vi "Message encoder.vi"(8 "error in (no error)":errorcluster, 10 "Data":variant, 11 "Kasli Writer in":refnum<class "Kasli Writer.lvclass">) -> (0 "error out":errorcluster, 2 "Message encoded":string, 3 "Kasli Writer out":refnum<class "Kasli Writer.lvclass">)   [LabVIEW 2020, in "CIRCUS_uServices.lvlib" / "Kasli Listener and Writer.lvlib" / "Kasli Writer.lvclass"]
uses:
  Kasli Writer.lvclass
  TALOS/TALOS_PPL.lvlibp
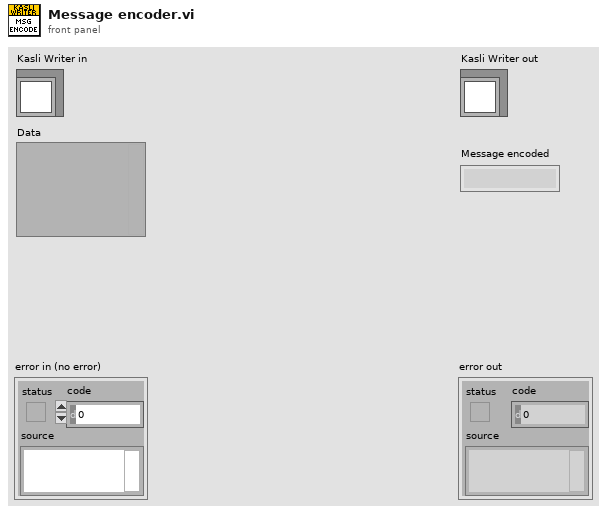
[diagram p1: front panel]
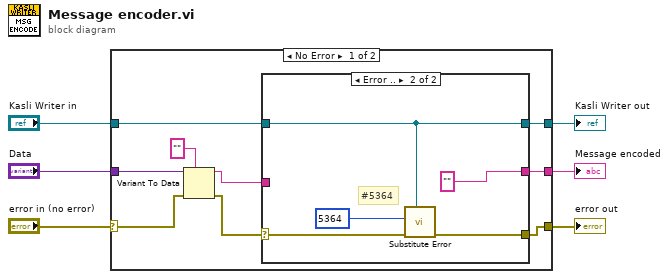
[diagram p0: block diagram]
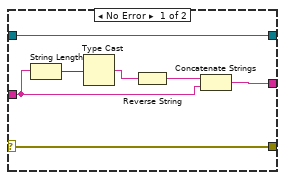
[diagram p2: hidden frame]
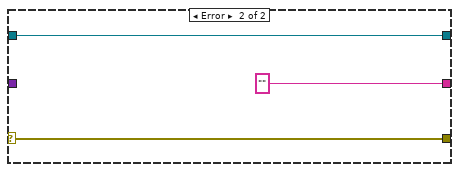
[diagram p3: hidden frame]
diagram:
  n1 = case shown="No Error" "error in (no error)" {
    selector: "error in (no error)" -> [w13 w28]
    tunnel: "Data" -> [w15 _]
    tunnel: [w7 ""] -> w5
    tunnel: [w8 w28] -> w3
    tunnel: "Kasli Writer in" -> [w12 w30]
    tunnel: [w11 w30] -> w1
    frame No Error {
      n2 = Variant To Data(error in=w13, type="", Variant=w15) -> (data=w10:string, error out=w9:errorcluster)
      n3 = case shown="Error .." w9 {
        selector: w9 -> [w18 w26]
        tunnel: [w22 w24] -> w11
        tunnel: w12 -> [w22 w24]
        tunnel: w10 -> [w20 _]
        tunnel: [w19 ""] -> w7
        tunnel: [w18 w25] -> w8
        frame No Error {
          n4 = String Length(string=w20) -> (length=w17:i32)
          n5 = Type Cast(x=w17) -> (*(type *) &x=w21:string)  [unwired: 1 in]
          n6 = Reverse String(1:w21) -> (0:w16:string)
          n7 = Concatenate Strings(w16, w20) -> (w19:string)
        }
        frame Error {
          # "#5364"
          n8 = call "Substitute Error.vi"("LabVIEW Object"=w24, "error in (no error)"=w26, "Error Code"=5364) -> ("error out"=w25:errorcluster)  [unwired: 8 in]
        }
      }
    }
    frame Error {
    }
  }
  "error out" <- w3
  "Kasli Writer out" <- w1
  "Message encoded" <- w5
